vi "Define.vi"(11 "Double Definition":T1) -> (3 "Double out":refnum<class "Double.lvclass">)   [LabVIEW 2020, in "Conditu2.lvlib" / "Columns.lvlib" / "Double.lvclass"]
uses:
  Double.lvclass
  C:/dev/lv20CE/lv-conditum-tools/Conditum-Clone/Columns/Type/Type.lvclass
  Double Definition.ctl
  Type/Definition.ctl
  Attributes.ctl
  Definition.ctl
  Field Type.ctl
  Type/Type.lvclass/Type.ctl
  Double.lvclass/Double.ctl
  Type/Type.lvclass
  Conditu2.lvlib
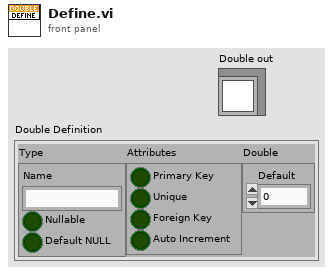
[diagram p1: front panel]
types:
  T1 = typedef "Conditu2.lvlib/Columns.lvlib/Double.lvclass/Double Definition.ctl" = cluster{"Type":T2, "Attributes":T3, "Double":T4}
  T2 = typedef "Conditu2.lvlib/Columns.lvlib/Type.lvclass/Definition.ctl" = cluster{"Name":string, "Nullable":bool, "Default NULL":bool}
  T3 = typedef "Conditu2.lvlib/Attributes.ctl" = cluster{"Primary Key":bool, "Unique":bool, "Foreign Key":bool, "Auto Increment":bool}
  T4 = typedef "Conditu2.lvlib/Columns.lvlib/Double.lvclass/Definition.ctl" = cluster{"Default":dbl}
  T5 = typedef "Conditu2.lvlib/Field Type.ctl" = enum16{"None", "ID", "Boolean", "Integer", "Double", "Timestamp", "String", "Text", "Entity"}
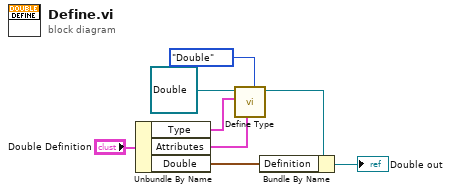
[diagram p0: block diagram]
diagram:
  n1 = Unbundle By Name("Double Definition") -> ("Type"=w6:T2, "Attributes"=w5:T3, "Double"=w4:T4)
  n2 = call "Define Type.vi"("Type"=Field_Type."Double", "Attributes"=w5, "Definition"=w6, "Type in"=refnum<class "Double.lvclass"> refnum ("Double in")) -> ("Type out"=w3:refnum<class "Double.lvclass">)  [unwired: 7 in]
  n3 = Bundle By Name(cluster=w3, "Definition"=w4) -> (→"Double out":refnum<class "Double.lvclass">)
